vi "TCP Initialize Server.vi"   [LabVIEW 2016, in "SLL Easy API via TCP.lvclass"]
doc: "Initialize the TCP Server."
uses:
  SLL Easy API via TCP.lvclass
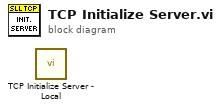
[diagram p0: block diagram]
diagram:
  n1 = call "TCP Initialize Server - Local.vi"() -> ()  [unwired: 9 in, 3 out]
